vi "Build_Write Multiple Holding Registers.vi"(8 "error in (no error)":errorcluster, 9 "values":u16[](array[numeric]), 10 "starting address":u16) -> (0 "error out":errorcluster, 3 "MB_PDU":T1={"Function Code"=1, "Data"=[], "RTU_DataBytes"=0})   [LabVIEW 2021, in "MB Master.lvlib"]
doc: "Builds PDU for Write Multiple Registers (function code 16)."
uses:
  <vilib>/Plasmionique/MB Master/MB Master.lvlib
  <vilib>/Plasmionique/MB Master/MB_PDU/MB_PDU_Cluster.ctl
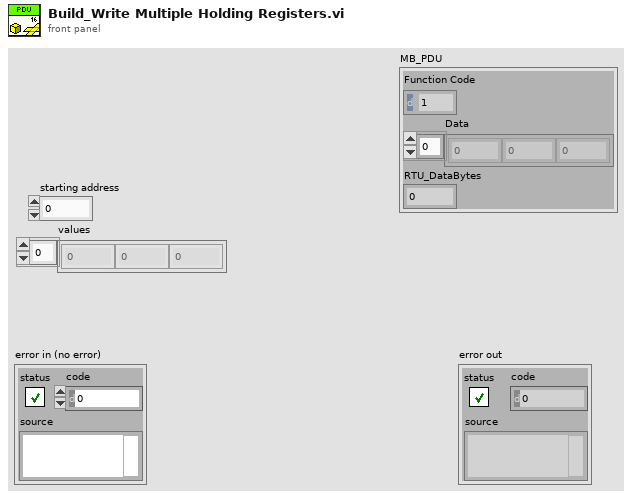
[diagram p1: front panel]
types:
  T1 = typedef "MB Master.lvlib/MB_PDU_Cluster.ctl" = cluster{"Function Code":u8, "Data":u8[], "RTU_DataBytes":i32}
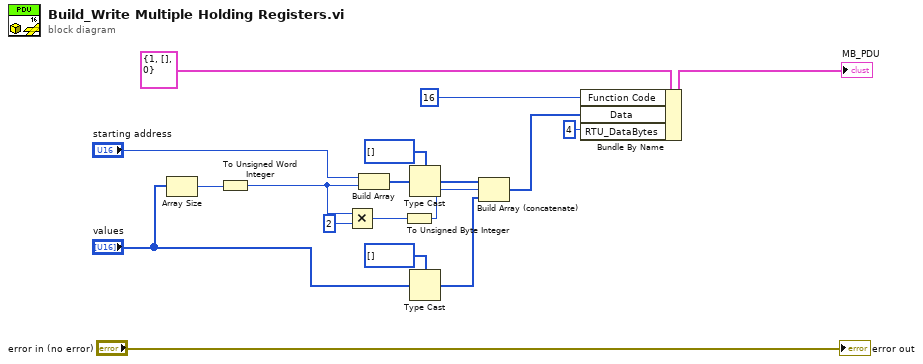
[diagram p0: block diagram]
diagram:
  n1 = Array Size(array="values") -> (size(s)=w3:i32)
  n2 = To Unsigned Word Integer(number=w3) -> (unsigned 16bit integer=w2:u16)
  n3 = Multiply(x=w2, y=u16 2) -> (x*y=w10:u16)
  n4 = Build Array("starting address", w2) -> (w18:u16[])
  n5 = To Unsigned Byte Integer(number=w10) -> (unsigned 8bit integer=w8:u8)
  n6 = Type Cast(type=u8[] [], x=w18) -> (*(type *) &x=w9:u8[])
  n7 = Type Cast(type=u8[] [], x="values") -> (*(type *) &x=w6:u8[])
  n8 = Build Array (concatenate)(w9, w8, w6) -> (w5:u8[])
  n9 = Bundle By Name(cluster=T1 {"Function Code"=1, "Data"=[], "RTU_DataBytes"=0} ("Modbus Serial New.lvlib:MB_PDU.lvclass"), "Function Code"=u8 16, "Data"=w5, "RTU_DataBytes"=4 ("NumBytes")) -> (→"MB_PDU":T1)
  "error out" <- "error in (no error)"
